vi "Set Sorting Format.vi"(8 "error in (no error)":errorcluster caption="错误输入（无错误）", 10 "Sorting":i32(ring) items=["None", "Ascending", "Descending"], 11 "ListViewClass 输入":refnum<class "ListViewClass.lvclass"> caption="DNL_LabVIEW Object in") -> (0 "error out":errorcluster caption="错误输出", 3 "ListViewClass 输出":refnum<class "ListViewClass.lvclass"> caption="DNL_LabVIEW Object out")   [LabVIEW 2012, in "ListViewClass.lvclass"]
uses:
  ListViewClass.lvclass
  ListViewClass.lvclass/ListViewClass.ctl
  System.Windows.Forms
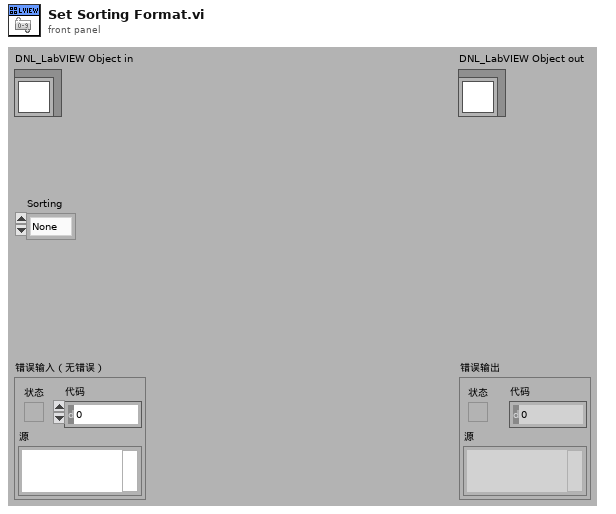
[diagram p1: front panel]
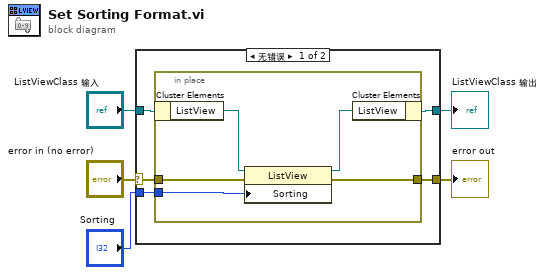
[diagram p0: block diagram]
diagram:
  n1 = case shown="无错误" "error in (no error)" {
    selector: "error in (no error)" -> [w8 w17]
    tunnel: [w7 w17] -> w4
    tunnel: [w6 w16] -> w2
    tunnel: "ListViewClass 输入" -> [w10 w16]
    tunnel: "Sorting" -> [w9 _]
    frame No Error {
      n2 = in-place {
        in-place-border: w9 -> [w15]
        in-place-border: w8 -> [w12]
        in-place-border: [w11] -> w7
        n3 = in-place-cluster #1(w10) -> ("ListView"=w14:refnum<k24>)
        n4 = property class="ListView"(reference=w14, error in=w12, "Sorting"=w15) -> (reference out=w13:refnum<k24>, error out=w11:errorcluster)
        n5 = in-place-cluster #1("ListView"=w13) -> (w6:refnum<class "ListViewClass.lvclass">)
      }
    }
    frame Error {
    }
  }
  "error out" <- w4
  "ListViewClass 输出" <- w2
